vi "Protect Unprotect.vi"() -> ()   [LabVIEW 2018]
doc: "©2019\nWiebe Walstra\nwww.carya.nl"
uses:
  System.Security
panel:
  out "string":string
  out "Protect":u8[](array[numeric])
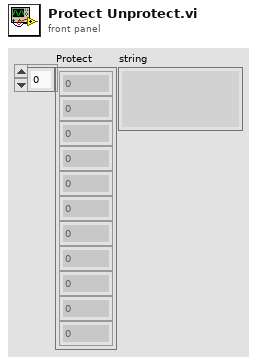
[diagram p1: front panel]
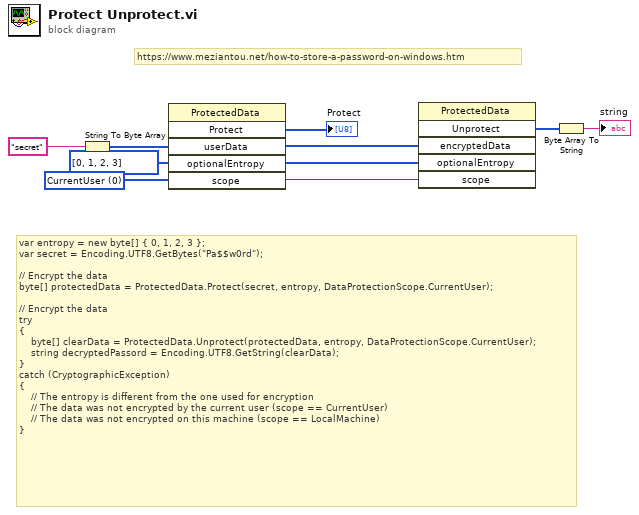
[diagram p0: block diagram]
diagram:
  w3 = 0 items=["CurrentUser", "LocalMachine"] ("scope")
  # "https://www.meziantou.net/how-to-store-a-password-on-windows.htm"
  # "var entropy = new byte[] { 0, 1, 2, 3 };\nvar secret = Encoding.UTF8.GetBytes(\"Pa$$w0rd\");\n\n// Encrypt the data\nbyte[] protectedData = ProtectedData.Protect(secret, entropy, DataProtectionScope.CurrentUser);\n\n// Encrypt the data\ntry\n{\n    byte[] clearData = ProtectedData.Unprotect(protectedData, entropy, DataProtectionScope.CurrentUser);\n    string decryptedPassord = Encoding.UTF8.GetString(clearData);\n}\ncatch (CryptographicException)\n{\n    // The entropy is different from the one used for encryption\n    // The data was not encrypted by the current user (scope == CurrentUser)\n    // The data was not encrypted on this machine (scope == LocalMachine)\n}"
  n1 = String To Byte Array(string="secret") -> (unsigned byte array=w7:u8[])
  n2 = invoke class="ProtectedData" method="Protect"("userData"=w7, "optionalEntropy"=u8[] [0, 1, 2, 3], "scope"=w3) -> ("Protect"=w5:u8[], "optionalEntropy"=w4:u8[])  [unwired: 3 in, 4 out]
  "Protect" <- w5
  n3 = invoke class="ProtectedData" method="Unprotect"("encryptedData"=w5, "optionalEntropy"=w4, "scope"=w3) -> ("Unprotect"=w2:u8[])  [unwired: 3 in, 5 out]
  n4 = Byte Array To String(unsigned byte array=w2) -> (string=→"string":string)
